vi "VISA Write-Read.vi"(7 "Max bytes to read":u32=4096, 8 "error in (no error)":errorcluster, 9 "Command String":string, 10 "Action":enum16{"Write", "Read", "Write & Read"}(ring)=enum."Write & Read", 11 "PS Driver.lvlib:PS Driver AMI4xx.lvclass":refnum<class "PS Driver AMI4xx.lvclass">) -> (0 "error out":errorcluster, 1 "Timeout?":bool, 2 "Response string":string, 3 "PS Driver.lvlib:PS Driver AMI4xx.lvclass out":refnum<class "PS Driver AMI4xx.lvclass">)   [LabVIEW 2025, in "PS Driver.lvlib" / "PS Driver AMI4xx.lvclass"]
doc: "Author: Scott Hannahs <sth@magnet.fsu.edu>\n\nThis software is licensed for use under the “MIT License\"\nCopyright (c) 2025 Scott Hannahs, sth@sth@magnet.sthnet.net\n\nPermission is hereby granted, free of charge, to any person obtaining a copy of this software and associated documentation files (the \"Software\"), to deal in the Software without restriction, including without limitation the rights to use, copy, modify, merge, publish, distribute, sublicense, and/or sell copies of the Software, and to permit persons to whom the Software is furnished to do so, subject to the following conditions: The above copyright notice and this permission notice shall be included in all copies or substantial portions of the Software.\n\nTHE SOFTWARE IS PROVIDED \"AS IS\", WITHOUT WARRANTY OF ANY KIND, EXPRESS OR IMPLIED, INCLUDING BUT NOT LIMITED TO THE WARRANTIES OF MERCHANTABILITY, FITNESS FOR A PARTICULAR PURPOSE AND NONINFRINGEMENT. IN NO EVENT SHALL THE AUTHORS OR COPYRIGHT HOLDERS BE LIABLE FOR ANY CLAIM, DAMAGES OR OTHER LIABILITY, WHETHER IN AN ACTION OF CONTRACT, TORT OR OTHERWISE, ARISING FROM, OUT OF OR IN CONNECTION WITH THE SOFTWARE OR THE USE OR OTHER DEALINGS IN THE SOFTWARE."
uses:
  AMI 4xx/PS Driver AMI4xx.lvclass
  PS Driver.lvclass/PS Driver.ctl
  PS Driver.lvclass
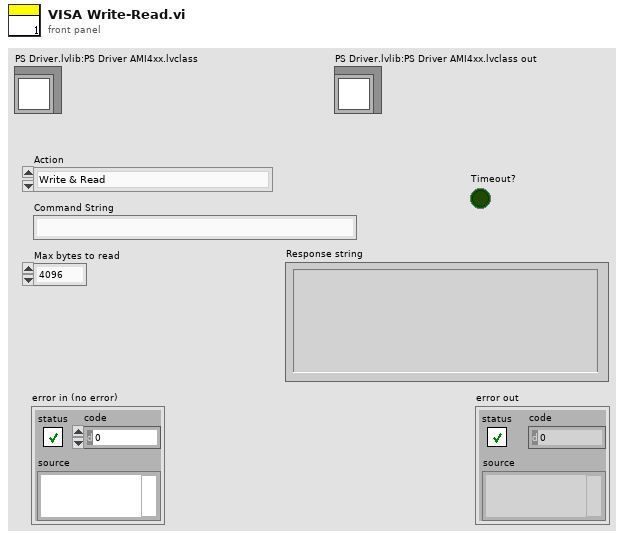
[diagram p1: front panel]
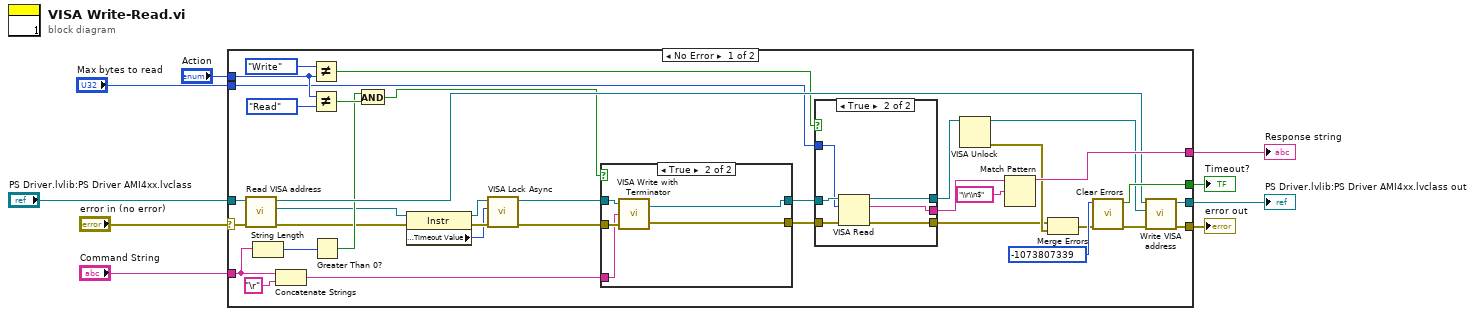
[diagram p0: block diagram]
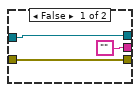
[diagram p2: hidden frame]
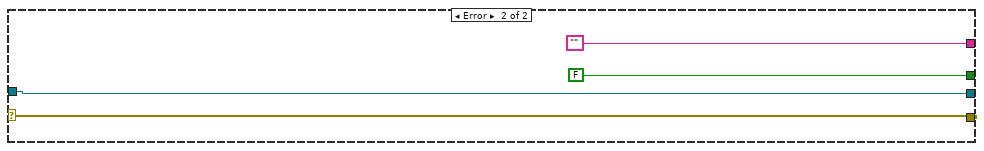
[diagram p4: hidden frame]
diagram:
  n1 = case shown="No Error" "error in (no error)" {
    selector: "error in (no error)" -> [w41 w66]
    tunnel: [w38 w66] -> w8
    tunnel: [w37 w65] -> w7
    tunnel: "PS Driver.lvlib:PS Driver AMI4xx.lvclass" -> [w40 w65]
    tunnel: [w43 ""] -> w6
    tunnel: "Command String" -> [w30 _]
    tunnel: "Action" -> [w28 _]
    tunnel: [w42 FALSE] -> w3
    tunnel: "Max bytes to read" -> [w13 _]
    frame No Error {
      n2 = call "Read VISA address.vi"("error in (no error)"=w41, "PS Driver in"=w40) -> ("error out"=w26:errorcluster, "VISA address"=w27:refnum<visa-resource-name>, "PS Driver out"=w36:refnum<class "PS Driver AMI4xx.lvclass">)  [unwired: 7 in]
      n3 = String Length(string=w30) -> (length=w33:i32)
      n4 = Concatenate Strings(w30, "\r") -> (w20:string)
      n5 = Not Equal?(x=enum16{"Write", "Read", "Write & Read"}."Write" ("y"), y=w28) -> (x != y?=w19:bool)
      n6 = Not Equal?(x=w28, y=enum16{"Write", "Read", "Write & Read"}."Read") -> (x != y?=w34:bool)
      n7 = Greater Than 0?(x=w33) -> (x > 0?=w32:bool)
      n8 = And(x=w32, y=w34) -> (x .and. y?=w29:bool)
      n9 = property class="Instr"(reference=w27, error in=w26) -> (reference out=w25:refnum<visa-resource-name>, error out=w24:errorcluster, "General Settings:Timeout Value"=w23:u32)
      n10 = call <vilib>:"VISA Lock Async.vi"("error in (no error)"=w24, "timeout (0)"=w23, "VISA resource name"=w25) -> ("error out"=w21:errorcluster, "VISA resource name out"=w22:refnum<visa-resource-name>)  [unwired: 6 in, 1 out]
      n11 = case shown="True" w29 {
        tunnel: w22 -> [w57 w62]
        tunnel: w21 -> [w56 w61]
        tunnel: w20 -> [_ w60]
        tunnel: [w57 w59] -> w18
        tunnel: [w56 w58] -> w17
        frame False {
        }
        frame True {
          n12 = call "VISA Write with Terminator.vi"("error in (no error)"=w61, "String to Write"=w60, "VISA session"=w62) -> ("error out"=w58:errorcluster, "dup VISA session"=w59:refnum<visa-resource-name>)
        }
      }
      n13 = case shown="True" w19 {
        tunnel: w18 -> [w49 w55]
        tunnel: w17 -> [w48 w54]
        tunnel: [w49 w53] -> w16
        tunnel: [w48 w52] -> w11
        tunnel: ["" w51] -> w14
        tunnel: w13 -> [_ w50]
        frame False {
        }
        frame True {
          n14 = VISA Read(VISA resource name=w55, byte count=w50, error in (no error)=w54) -> (VISA resource name out=w53:refnum<visa-resource-name>, read buffer=w51:string, error out=w52:errorcluster)  [unwired: 1 out]
        }
      }
      n15 = VISA Unlock(11:w16) -> (0:w12:errorcluster, 3:w15:refnum<visa-resource-name>)  [unwired: 1 in]
      n16 = Match Pattern(string=w14, regular expression="\\r\\n$") -> (before substring=w43:string)  [unwired: 1 in, 3 out]
      n17 = Merge Errors(w11, w12) -> (w10:errorcluster)
      n18 = call <vilib>:"Clear Errors.vi"("error in (no error)"=w10, "specific error code to clear (0: all)"=-1073807339) -> ("error out"=w39:errorcluster, "specific error cleared?"=w42:bool)  [unwired: 4 in]
      n19 = call "Write VISA address.vi"("error in (no error)"=w39, "VISA address"=w15, "PS Driver in"=w36) -> ("error out"=w38:errorcluster, "PS Driver out"=w37:refnum<class "PS Driver AMI4xx.lvclass">)  [unwired: 7 in]
    }
    frame Error {
    }
  }
  "error out" <- w8
  "Response string" <- w6
  "Timeout?" <- w3
  "PS Driver.lvlib:PS Driver AMI4xx.lvclass out" <- w7
